vi "UTIL Compute Multivariate Probability.vi"(3 "Sigma":dbl[][](array[numeric]), 4 "Mu":dbl[](array[numeric]), 5 "Data Point":dbl[](array[numeric])) -> (1 "P(x,mu,sigma)":dbl)   [LabVIEW 2017]
doc: "This VI computes the probability of a data point belonging to a multivariate gaussian distribution with vector mean mu and covariance matrix Sigma.\n\nInputs\n Data Point 1-D Array of DBL\n Mu 1-D Array of DBL\n Sigma 2-D Array of DBL\n\nOutputs\n P(x,mu,sigma) DBL"
uses:
  <vilib>/Analysis/baseanly.llb/Matrix Type of Inverse Matrix.ctl
  <vilib>/Analysis/baseanly.llb/Real Determinant.vi
  <vilib>/Analysis/baseanly.llb/Vector x A.vi
  <vilib>/Analysis/baseanly.llb/Real Dot Product.vi
  <vilib>/Analysis/baseanly.llb/Real Inverse Matrix.vi
  <vilib>/Analysis/NI_AALBase.lvlib
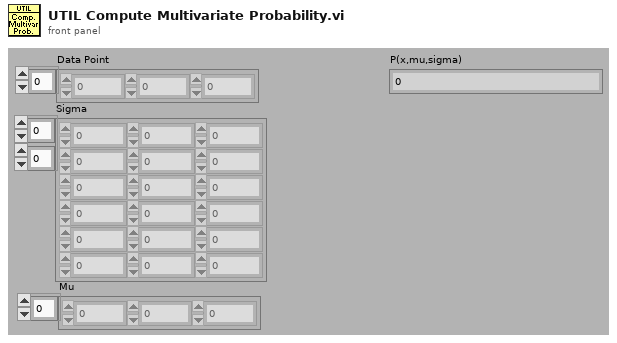
[diagram p1: front panel]
types:
  T1 = typedef "NI_AALBase.lvlib/Matrix Type of Inverse Matrix.ctl" = enum32{"General", "Positive Definite", "Lower Triangular", "Upper Triangular"}
  T2 = typedef "NI_Matrix.lvlib/RealMatrix.ctl" = dbl[][]
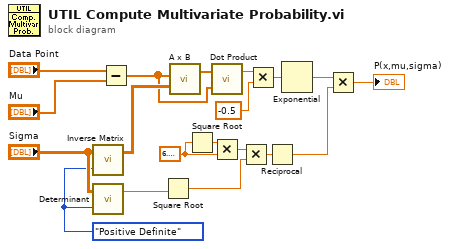
[diagram p0: block diagram]
diagram:
  w6 = Matrix_Type_of_Inverse_Matrix."Positive Definite" ("matrix type")
  w10 = 6.283185307179586
  n1 = call-poly <vilib>:"Inverse Matrix.vi"("matrix type"=w6, "Input Matrix"="Sigma") -> ("Inverse Matrix"=w17:T2)  [unwired: 1 out]
  n2 = call-poly <vilib>:"Determinant.vi"("matrix type"=w6, "Input Matrix"="Sigma") -> ("determinant"=w2:dbl)  [unwired: 1 out]
  n3 = Subtract(x="Data Point", y="Mu") -> (x-y=w15:dbl[])
  n4 = Square Root(x=w2) -> (sqrt(x)=w1:dbl)
  n5 = call-poly <vilib>:"A x B.vi"("Matrix A"=w17, "Vector V'"=w15) -> ("V' x A"=w16:dbl[])  [unwired: 1 out]
  n6 = Square Root(x=w10) -> (sqrt(x)=w9:dbl)
  n7 = call-poly <vilib>:"Dot Product.vi"("Y Vector"=w15, "X Vector"=w16) -> ("X * Y"=w13:dbl)  [unwired: 1 out]
  n8 = Multiply(x=w9, y=w10) -> (x*y=w11:dbl)
  n9 = Multiply(x=w11, y=w1) -> (x*y=w8:dbl)
  n10 = Multiply(x=w13, y=-0.5) -> (x*y=w12:dbl)
  n11 = Reciprocal(x=w8) -> (1/x=w4:dbl)
  n12 = Exponential(1:w12) -> (0:w5:dbl)
  n13 = Multiply(x=w5, y=w4) -> (x*y=→"P(x,mu,sigma)":dbl)
